vi "GAS_INLET_STAGE.vi"() -> (0 "Inlet Pressure":dbl(graph), 1 "Inlet Temperature":dbl(graph), 2 "Inlet Temperature Transmitter":dbl, 3 "Inlet Pressure Transmitter":dbl)   [LabVIEW 2014]
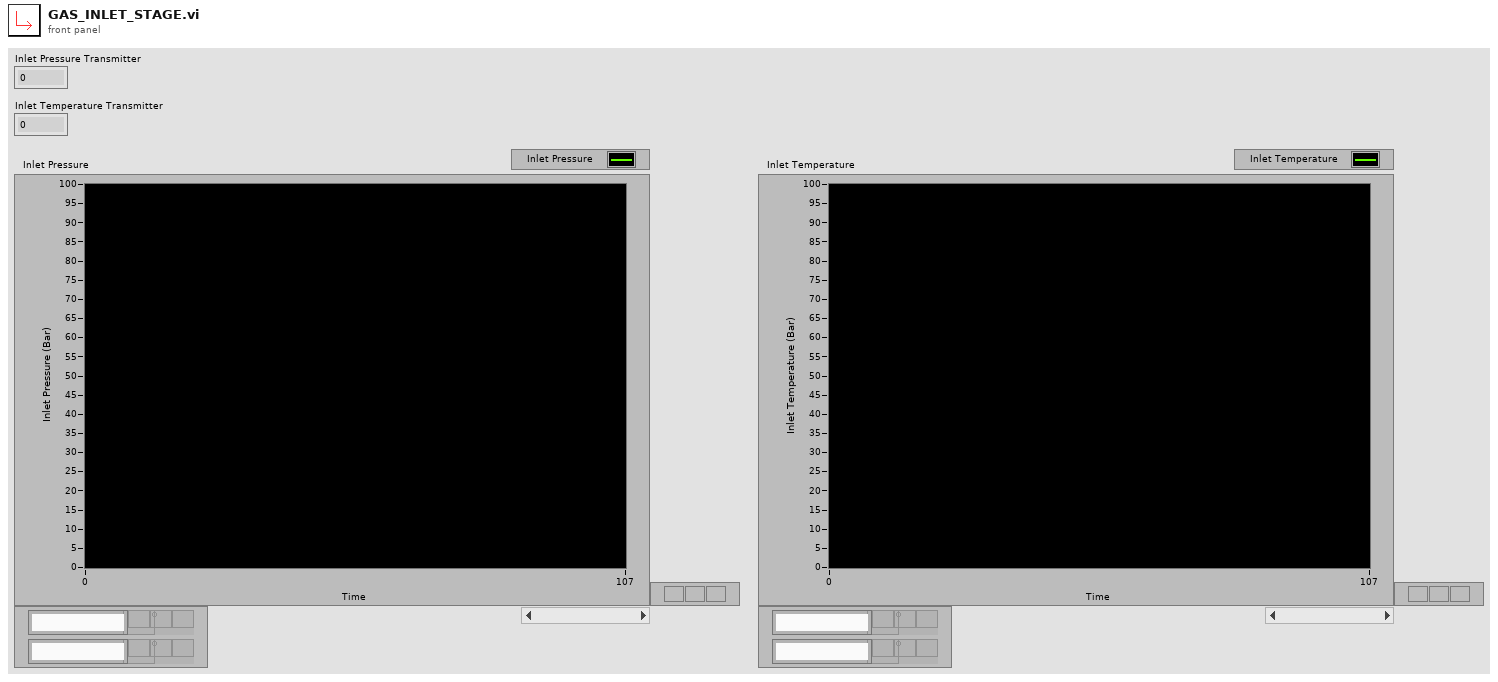
[diagram p1: front panel]
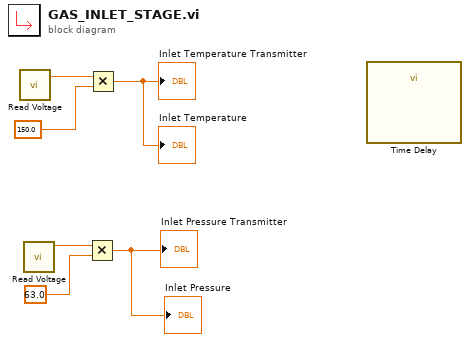
[diagram p0: block diagram]
diagram:
  n1 = call "Read Voltage.vi"() -> ("voltage"=w4:dbl)  [unwired: 6 in, 1 out]
  n2 = call "Read Voltage.vi"() -> ("voltage"=w6:dbl)  [unwired: 6 in, 1 out]
  n3 = Multiply(x=w6, y=63.0) -> (x*y=→"Inlet Pressure Transmitter" →"Inlet Pressure":dbl)
  n4 = Multiply(x=w4, y=150.0) -> (x*y=→"Inlet Temperature Transmitter" →"Inlet Temperature":dbl)
  n5 = call "Time Delay"() -> ()  [unwired: 11 in, 1 out]
